vi "Search.vi"(8 "error in (no error)":errorcluster, 10 "LLNode in":refnum<data-value>, 11 "LLSearch in":refnum<class "LLSearch.lvclass">) -> (0 "error out":errorcluster, 1 "found":bool, 2 "LLNode out":refnum<data-value>, 3 "LLSearch out":refnum<class "LLSearch.lvclass">)   [LabVIEW 2009, in "LLSearch.lvclass"]
uses:
  LLSearch.lvclass
  LLNode/LLNode.lvclass
  Node/Node.lvclass
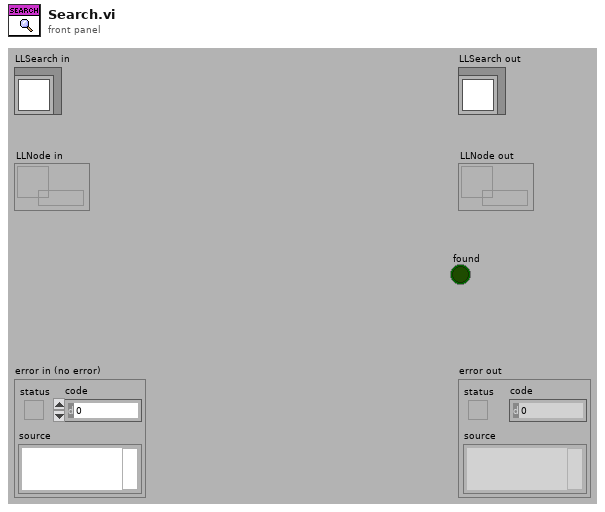
[diagram p1: front panel]
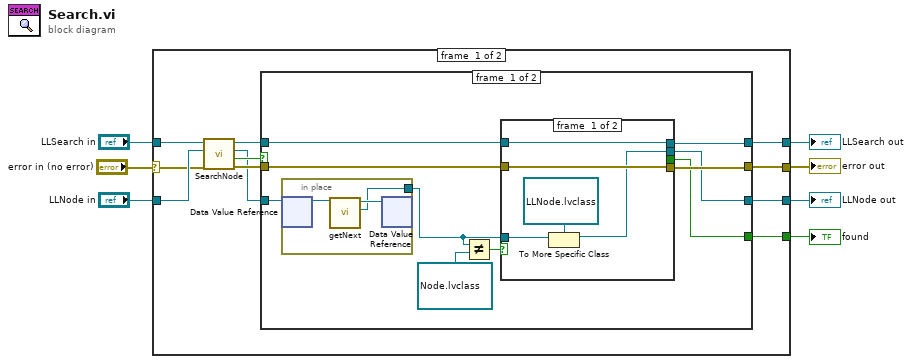
[diagram p0: block diagram]
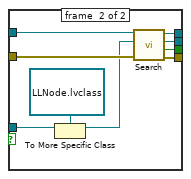
[diagram p2: hidden frame]
diagram:
  n1 = case shown="No Error" "error in (no error)" {
    selector: "error in (no error)" -> [w16 w50]
    tunnel: [w11 w52] -> w5
    tunnel: "LLSearch in" -> [w18 w52]
    tunnel: "LLNode in" -> [w17 w51]
    tunnel: [w8 w51] -> w3
    tunnel: [w9 _] -> w2
    tunnel: [w10 w50] -> w1
    frame #0 {
      n2 = call-dynamic "SearchNode.vi"("error in (no error)"=w16, "LLNode in"=w17, "LLSearch in"=w18) -> ("error out"=w14:errorcluster, "found"=w15:bool, "LLNode out"=w12:refnum<data-value>, "LLSearch out"=w13:refnum<class "LLSearch.lvclass">)  [unwired: 5 in]
      n3 = case shown="False" w15 {
        selector: w15 -> [_ w47]
        tunnel: w14 -> [w23 w48]
        tunnel: w13 -> [w27 w49]
        tunnel: w12 -> [w28 w46]
        tunnel: [w26 w49] -> w11
        tunnel: [w25 w48] -> w10
        tunnel: [w24 w47] -> w9
        tunnel: [w22 w46] -> w8
        frame #0 {
          n4 = in-place {
            in-place-border: [w43] -> w20
            n5 = in-place-dvr #1(w28) -> (w45:refnum<class "LLNode.lvclass">)  [unwired: 1 out]
            n6 = call "getNext.vi"("LLNode in"=w45) -> ("next"=w43:refnum<data-value>, "LLNode out"=w44:refnum<class "LLNode.lvclass">)  [unwired: 8 in, 1 out]
            n7 = in-place-dvr #1(w44) -> ()  [unwired: 2 out]
          }
          n8 = Not Equal?(x=w20, y=refnum<data-value> refnum ("x")) -> (x != y?=w19:bool)
          n9 = case shown="False" w19 {
            tunnel: w27 -> [w33 w42]
            tunnel: [w33 w41] -> w26
            tunnel: [w32 w40] -> w25
            tunnel: [_ w39] -> w24
            tunnel: w23 -> [w32 w38]
            tunnel: [w29 w35] -> w22
            tunnel: w20 -> [w30 w34]
            frame #0 {
              n10 = To More Specific Class(target class=refnum<data-value> refnum ("LLNode out"), reference=w30) -> (specific class reference=w29:refnum<data-value>)  [unwired: 1 in, 1 out]
            }
            frame #1 {
              n11 = To More Specific Class(target class=refnum<data-value> refnum ("LLNode out"), reference=w34) -> (specific class reference=w36:refnum<data-value>)  [unwired: 1 in, 1 out]
              n12 = call "Search.vi"("error in (no error)"=w38, "LLNode in"=w36, "LLSearch in"=w42) -> ("error out"=w40:errorcluster, "found"=w39:bool, "LLNode out"=w35:refnum<data-value>, "LLSearch out"=w41:refnum<class "LLSearch.lvclass">)  [unwired: 5 in]
            }
          }
        }
        frame #1 {
        }
      }
    }
    frame #1 {
    }
  }
  "error out" <- w1
  "LLSearch out" <- w5
  "LLNode out" <- w3
  "found" <- w2
